vi "dispense2electricboogaloo.vi"(1 "NXT/EV3":T1, 5 "0-Blue Large":dbl, 7 "1-Red Large":dbl, 9 "2-Blue Small":dbl, 11 "3-Red Small":dbl, 12 "4-HDPE":dbl, 13 "5-Steel":dbl, 14 "6-White Large":dbl, 15 "7-White Small":dbl) -> (3 "NXT/EV3 2":T1)   [LabVIEW 2016]
uses:
  <vilib>/NXT/Subs/LVHSConnector.ctl
  <vilib>/NXT/LegoClasses/BrickReference/BrickReference.lvclass
  <vilib>/NXT/Block Support/NXT_OutputPort.ctl
  <vilib>/NXT/NXTIO Xnodes/NXTIONodeSubVIs/NXTMotorRunDistance.vi
  <vilib>/NXT/Dual Mode Library/Waits/Wait_Num.vi
  <vilib>/NXT/NXTIO Xnodes/AddressXNode/NXTIOAddress.xnode
  <vilib>/NXT/NXTIO Xnodes/NXTIOXNode/NXTIO.xnode
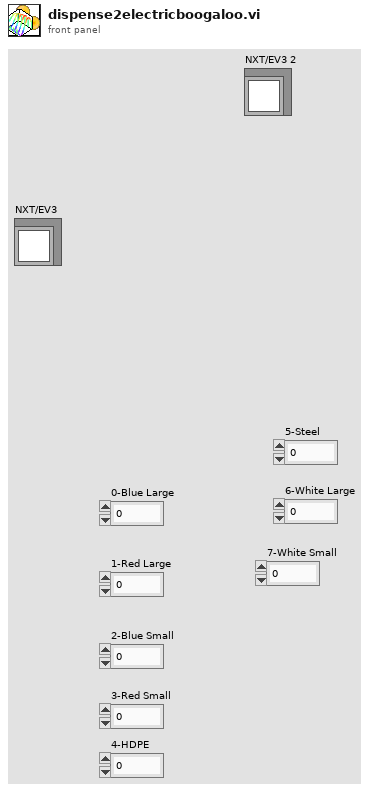
[diagram p1: front panel]
types:
  T1 = typedef "LVHSConnector.ctl" = refnum<class "BrickReference.lvclass">
  T2 = typedef "NXT_OutputPort.ctl" = u8
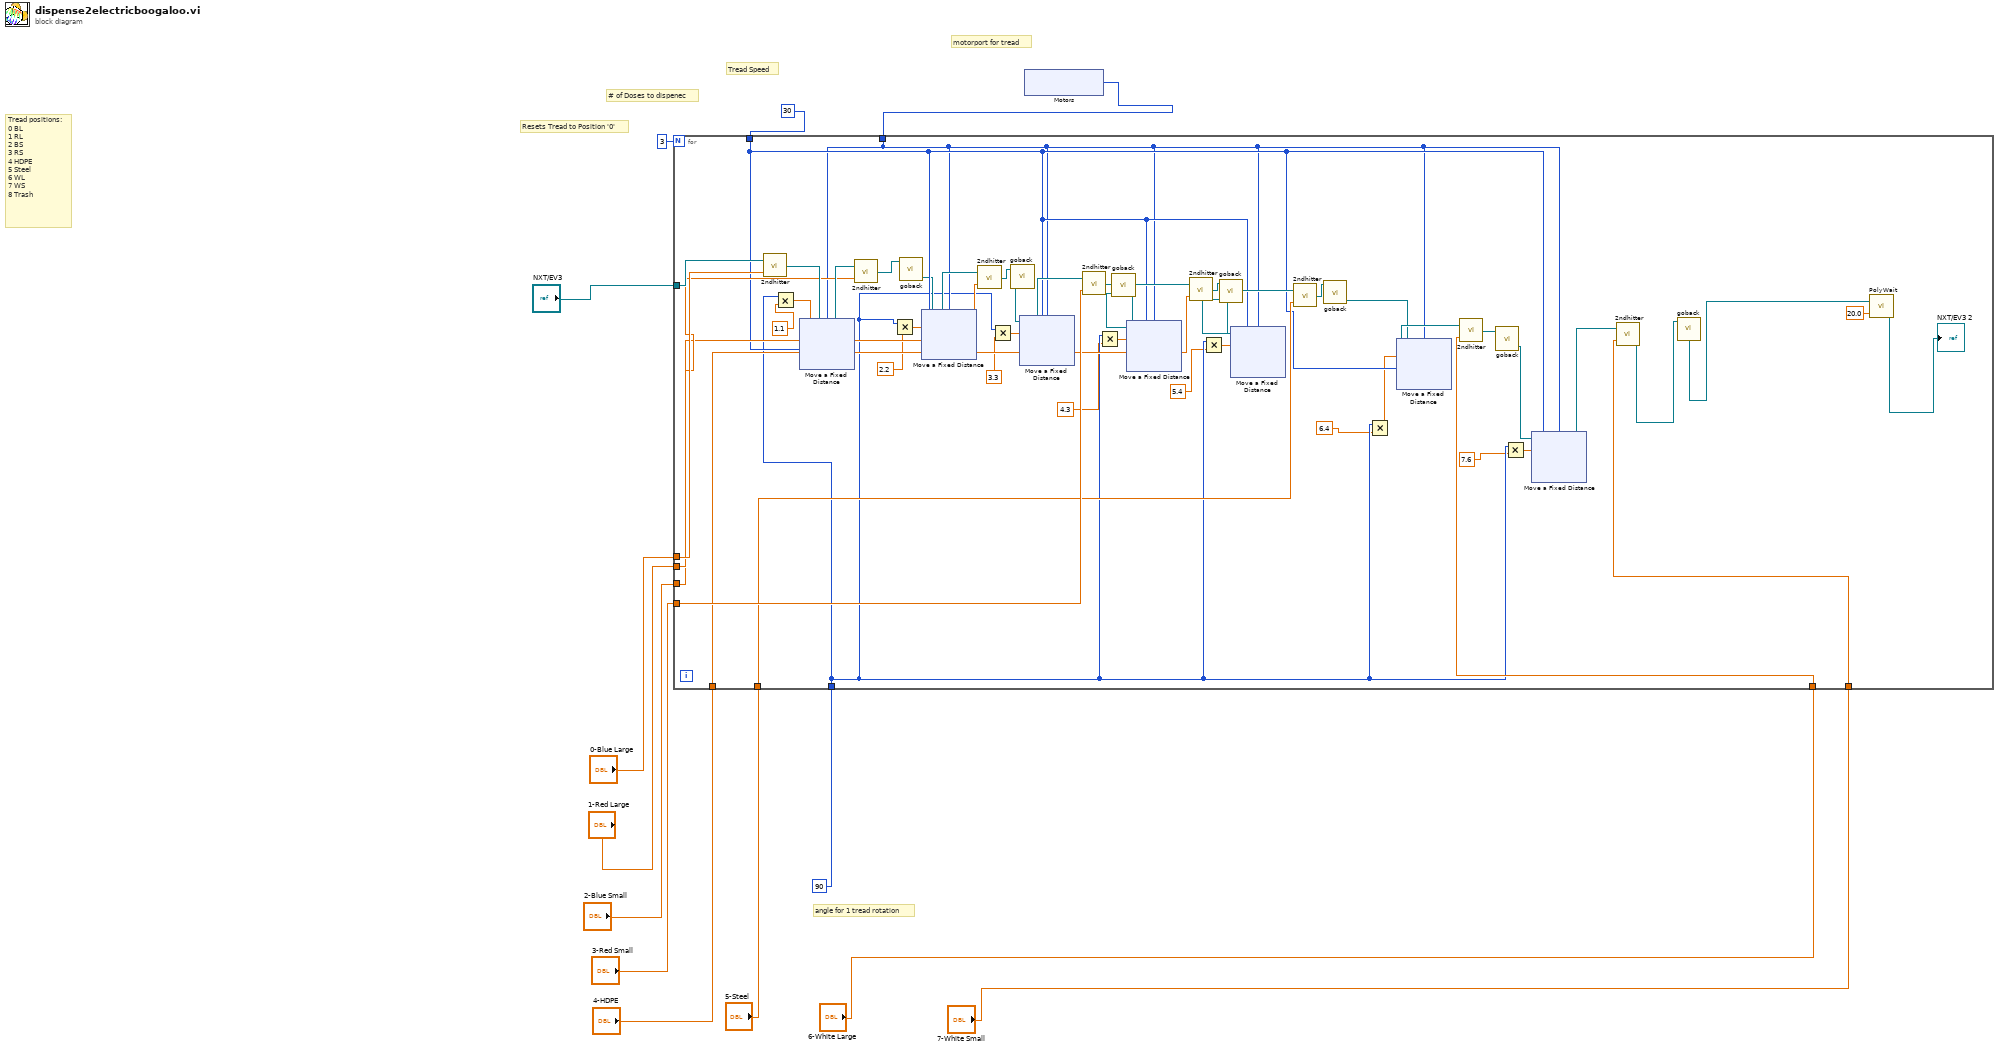
[diagram p0: block diagram]
diagram:
  # "angle for 1 tread rotation"
  # "Tread Speed"
  # "motorport for tread"
  # "# of Doses to dispenec"
  # "Resets Tread to Position '0'"
  # "Tread positions:\n0 BL\n1 RL\n2 BS\n3 RS\n4 HDPE\n5 Steel\n6 WL\n7 WS\n8 Trash"
  n1 = xnode "Motors"() -> ("Motor"=w11:T2)
  n2 = for {
    N: 3 -> [_]
    tunnel: "NXT/EV3" -> [w63]
    tunnel: "0-Blue Large" -> [w62]
    tunnel: w11 -> [w45]
    tunnel: 30 -> [w46]
    tunnel: "1-Red Large" -> [w59]
    tunnel: "2-Blue Small" -> [w57]
    tunnel: "3-Red Small" -> [w55]
    tunnel: "4-HDPE" -> [w53]
    tunnel: "5-Steel" -> [w51]
    tunnel: "6-White Large" -> [w49]
    tunnel: "7-White Small" -> [w47]
    tunnel: 90 -> [w21]
    n3 = call "2ndhitter.vi"("Marble Req"=w62, "NXT/EV3"=w63) -> ("NXT/EV3 2"=w61:T1)  [unwired: 1 in]
    n4 = Multiply(x=w21, y=1.1) -> (x*y=w28:dbl)
    n5 = xnode "Move a Fixed Distance"("Speed 1"=w46, "Distance 1"=w28, "Motors"=w45, "NXT/EV3"=w61) -> ("NXT/EV3"=w60:T1)
    n6 = call "2ndhitter.vi"("Marble Req"=w59, "NXT/EV3"=w60) -> ("NXT/EV3 2"=w42:T1)  [unwired: 1 in]
    n7 = Multiply(x=w21, y=2.2) -> (x*y=w27:dbl)
    n8 = call "goback.vi"("NXT/EV3"=w42) -> ("NXT/EV3 2"=w41:T1)  [unwired: 1 in]
    n9 = xnode "Move a Fixed Distance"("Speed 1"=w46, "Distance 1"=w27, "Motors"=w45, "NXT/EV3"=w41) -> ("NXT/EV3"=w58:T1)
    n10 = call "2ndhitter.vi"("Marble Req"=w57, "NXT/EV3"=w58) -> ("NXT/EV3 2"=w40:T1)  [unwired: 1 in]
    n11 = Multiply(x=w21, y=3.3) -> (x*y=w26:dbl)
    n12 = call "goback.vi"("NXT/EV3"=w40) -> ("NXT/EV3 2"=w39:T1)  [unwired: 1 in]
    n13 = xnode "Move a Fixed Distance"("Speed 1"=w46, "Distance 1"=w26, "Motors"=w45, "NXT/EV3"=w39) -> ("NXT/EV3"=w56:T1)
    n14 = call "2ndhitter.vi"("Marble Req"=w55, "NXT/EV3"=w56) -> ("NXT/EV3 2"=w38:T1)  [unwired: 1 in]
    n15 = Multiply(x=w21, y=4.3) -> (x*y=w25:dbl)
    n16 = call "goback.vi"("NXT/EV3"=w38) -> ("NXT/EV3 2"=w37:T1)  [unwired: 1 in]
    n17 = xnode "Move a Fixed Distance"("Speed 1"=w46, "Distance 1"=w25, "Motors"=w45, "NXT/EV3"=w37) -> ("NXT/EV3"=w54:T1)
    n18 = call "2ndhitter.vi"("Marble Req"=w53, "NXT/EV3"=w54) -> ("NXT/EV3 2"=w36:T1)  [unwired: 1 in]
    n19 = Multiply(x=w21, y=5.4) -> (x*y=w24:dbl)
    n20 = call "goback.vi"("NXT/EV3"=w36) -> ("NXT/EV3 2"=w35:T1)  [unwired: 1 in]
    n21 = xnode "Move a Fixed Distance"("Speed 1"=w46, "Distance 1"=w24, "Motors"=w45, "NXT/EV3"=w35) -> ("NXT/EV3"=w52:T1)
    n22 = call "2ndhitter.vi"("Marble Req"=w51, "NXT/EV3"=w52) -> ("NXT/EV3 2"=w34:T1)  [unwired: 1 in]
    n23 = call "goback.vi"("NXT/EV3"=w34) -> ("NXT/EV3 2"=w33:T1)  [unwired: 1 in]
    n24 = Multiply(x=w21, y=6.4) -> (x*y=w23:dbl)
    n25 = xnode "Move a Fixed Distance"("Speed 1"=w46, "Distance 1"=w23, "Motors"=w45, "NXT/EV3"=w33) -> ("NXT/EV3"=w50:T1)
    n26 = call "2ndhitter.vi"("Marble Req"=w49, "NXT/EV3"=w50) -> ("NXT/EV3 2"=w32:T1)  [unwired: 1 in]
    n27 = call "goback.vi"("NXT/EV3"=w32) -> ("NXT/EV3 2"=w31:T1)  [unwired: 1 in]
    n28 = Multiply(x=w21, y=7.6) -> (x*y=w22:dbl)
    n29 = xnode "Move a Fixed Distance"("Speed 1"=w46, "Distance 1"=w22, "Motors"=w45, "NXT/EV3"=w31) -> ("NXT/EV3"=w48:T1)
    n30 = call "2ndhitter.vi"("Marble Req"=w47, "NXT/EV3"=w48) -> ("NXT/EV3 2"=w30:T1)  [unwired: 1 in]
    n31 = call "goback.vi"("NXT/EV3"=w30) -> ("NXT/EV3 2"=w29:T1)  [unwired: 1 in]
    n32 = call-poly <vilib>:"PolyWait.vi"("Time (1 sec)"=sgl 20.0, "NXT/EV3"=w29) -> ("NXT/EV3"=→"NXT/EV3 2":T1)  [unwired: 2 in]
  }
